vi "Voltage-zero.vi"(8 "error in":errorcluster, 11 "VISA resource in":refnum<visa-resource-name>) -> (0 "error out":errorcluster, 3 "VISA resource out":refnum<visa-resource-name>)   [LabVIEW 2012]
uses:
  <instrlib>/Tektronix PWS4XXX Series/Tektronix PWS4XXX Series.lvlib
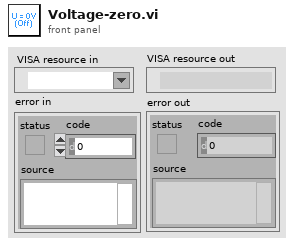
[diagram p1: front panel]
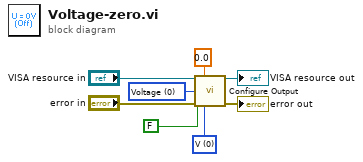
[diagram p0: block diagram]
diagram:
  w6 = u16 0 items=["V", "mV", "kV", "A", "mA"] ("Unit(V)")
  w7 = u16 0 items=["Voltage", "Current"] ("Function(0:Voltage)")
  n1 = call <instrlib>:"Configure Output.vi"("VISA resource name"="VISA resource in", "Manual Range(0.00)"=0.0, "Function(0:Voltage)"=w7, "Enable Output (T: Enable)"=FALSE, "error in (no error)"="error in", "Unit(V)"=w6) -> ("VISA resource name out"=→"VISA resource out":refnum<visa-resource-name>, "error out"=→"error out":errorcluster)  [unwired: 8 in]
